vi "Read TypeFirmware.vi"(8 "error in (no error)":errorcluster, 11 "ParameterConf in":refnum<class "ParameterConf.lvclass">) -> (0 "error out":errorcluster, 2 "TypeFirmware":T1, 3 "ParameterConf out":refnum<class "ParameterConf.lvclass">)   [LabVIEW 2017, in "LibraryGcode.lvlib" / "ParameterConf.lvclass"]
uses:
  ParameterConf.lvclass
  Firmware.ctl
  ParameterConf.lvclass/ParameterConf.ctl
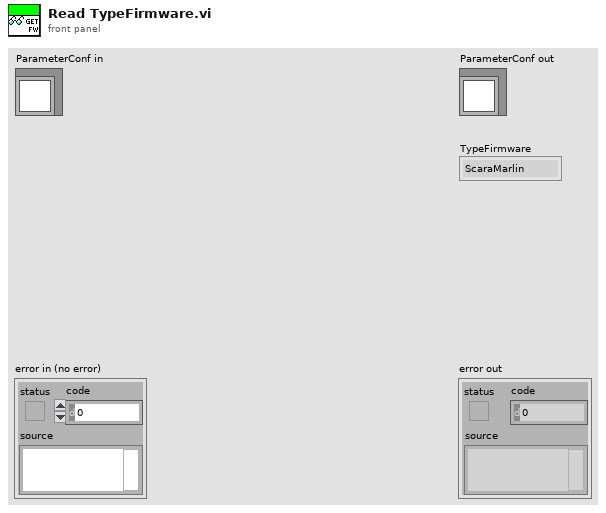
[diagram p1: front panel]
types:
  T1 = typedef "LibraryGcode.lvlib/ParameterConf.lvclass/Firmware.ctl" = enum16{"ScaraMarlin", "CncMarlin", "Mk4Due"}
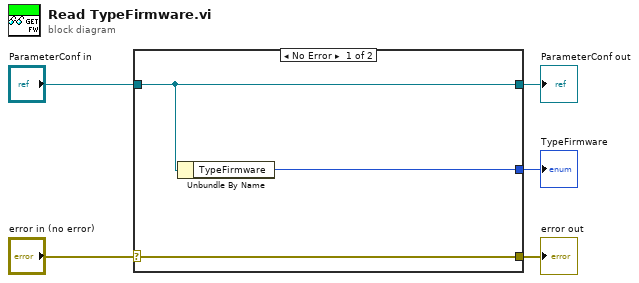
[diagram p0: block diagram]
diagram:
  n1 = case shown="No Error" "error in (no error)" {
    selector: "error in (no error)" -> [w8 w9]
    tunnel: [w8 w9] -> w4
    tunnel: [w7 w10] -> w2
    tunnel: "ParameterConf in" -> [w7 w10]
    tunnel: [w6 _] -> w1
    frame No Error {
      n2 = Unbundle By Name(w7) -> ("TypeFirmware"=w6:T1)
    }
    frame Error {
    }
  }
  "error out" <- w4
  "ParameterConf out" <- w2
  "TypeFirmware" <- w1
